vi "Test Fail on Unexpected Element in Array.vi"(8 "error in (no error)":errorcluster, 11 "LUnit Test Case V2 Test Double In":refnum<class "Test Case Test Double.lvclass">) -> (0 "error out":errorcluster, 3 "LUnit Test Case V2 Test Double Out":refnum<class "Test Case Test Double.lvclass">)   [LabVIEW 2020, in "Test Case Test Double.lvclass"]
uses:
  Test Case Test Double.lvclass
  fa902765-ef05-455b-87d3-fc84014acdc3.vi
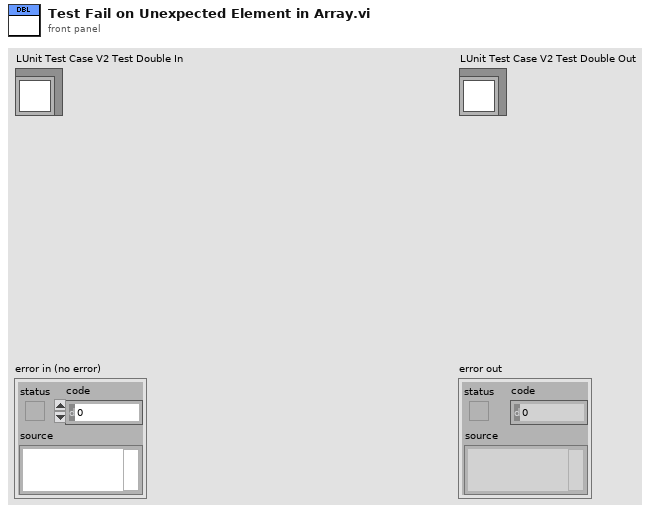
[diagram p1: front panel]
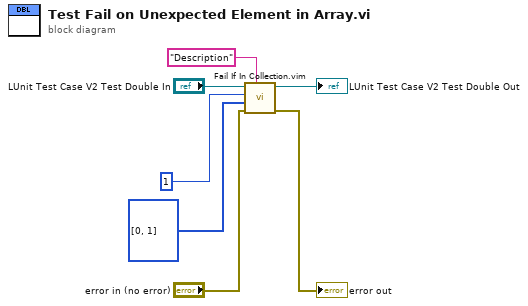
[diagram p0: block diagram]
diagram:
  n1 = call "Fail If In Collection.vim"("Description"="Description", "error in (no error)"="error in (no error)", "Collection"=i32[] [0, 1], "Element"=1, "LUnit Test Case In"="LUnit Test Case V2 Test Double In") -> ("error out"=→"error out":errorcluster, "LUnit Test Case Out"=→"LUnit Test Case V2 Test Double Out":refnum<class "Test Case Test Double.lvclass">)  [unwired: 5 in]
